vi "F Dwf Analog In Status Record.vi"(7 "pcdDataCorrupt":i32, 8 "error in (no error)":errorcluster, 9 "pcdDataLost":i32, 10 "pcdDataAvailable":i32, 11 "hdwf":i32) -> (0 "error out":errorcluster, 1 "pcdDataLost out":i32, 2 "pcdDataAvailable out":i32, 3 "function return":i32, 5 "pcdDataCorrupt out":i32)   [LabVIEW 2024, in "Olasdwf.lvlib"]
doc: "DWFAPI int FDwfAnalogInStatusRecord(HDWF hdwf, int *pcdDataAvailable, int *pcdDataLost, int *pcdDataCorrupt);"
uses:
  Olasdwf.lvlib
  Windows/System32/dwf.dll
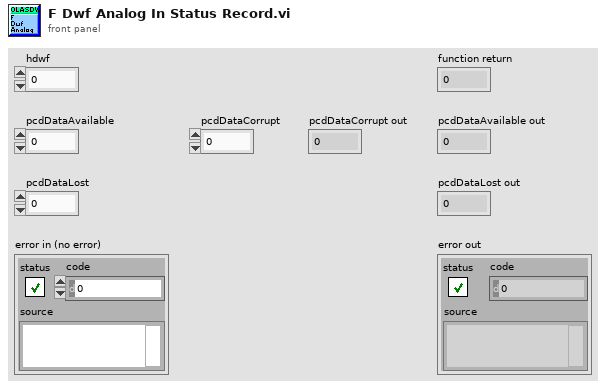
[diagram p1: front panel]
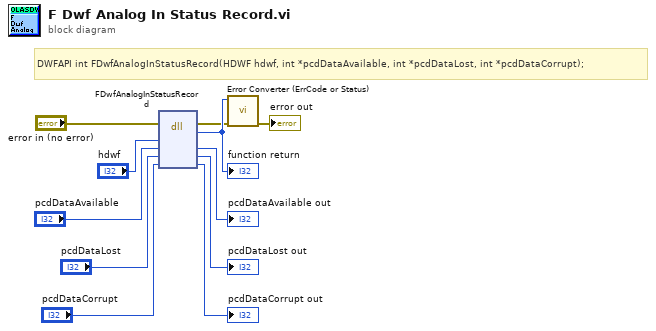
[diagram p0: block diagram]
diagram:
  # "DWFAPI int FDwfAnalogInStatusRecord(HDWF hdwf, int *pcdDataAvailable, int *pcdDataLost, int *pcdDataCorrupt);"
  n1 = dll-call lib="/Windows/System32/dwf.*" fn="FDwfAnalogInStatusRecord"(error in="error in (no error)", "hdwf"="hdwf", "pcdDataAvailable"="pcdDataAvailable", "pcdDataLost"="pcdDataLost", "pcdDataCorrupt"="pcdDataCorrupt") -> (error out=w2:errorcluster, w11:i32, "pcdDataAvailable"=→"pcdDataAvailable out":i32, "pcdDataLost"=→"pcdDataLost out":i32, "pcdDataCorrupt"=→"pcdDataCorrupt out":i32)  [unwired: 3 in, 1 out]
  "function return" <- w11
  n2 = call "Error Converter (ErrCode or Status).vi"("error in (no error)"=w2, "error code"=w11) -> ("error out"=→"error out":errorcluster)  [unwired: 9 in]
